vi "Import - Buffered Rx Packet.vi"(7 "Rx Packet":T2 {"targetPriority" min=-2 max=16 step=1; "targetProcessor" min=-2 max=16 step=1; "Endianness" items=["big-endian"=0, "little-endian"=2]}, 8 "error in (no error)":errorcluster, 11 "Device Item Ref in":T1 format="%.0x") -> (0 "error out":errorcluster, 3 "Device Item Ref out":T1 format="%.0x")   [LabVIEW 2019, in "UDP-Custom-Device System Explorer.lvlib"]
uses:
  UDP-Custom-Device System Explorer.lvlib
  <vilib>/NI VeriStand/Custom Device API/Custom Device Item Ref.ctl
  Types/XML - New/ImpExp - Rx Packet Data.ctl
  <vilib>/NI VeriStand/Custom Device API/Custom Device Item Info.ctl
  Shared/Types/Shared - Channel Data Type.ctl
  Shared/Types/Shared - Buffered.PacketInfo.ctl
  Shared/Types/Shared - Pointer Encoding.ctl
  Shared/Types/Shared - Receive Buffer Options.ctl
  Shared/Types/Shared - Transmit Buffer Options.ctl
  Shared/Types/Shared - New Data Options.ctl
  Shared/Types/Shared - Thread Management.ctl
  Property Accessors/Shared Packet Accessors.lvlib
  Property Accessors/Rx Packet Accessors.lvlib
  <vilib>/NI VeriStand/Custom Device API/Custom Device API.lvlib
  Property Accessors/Buffered Data Packet.lvlib
  Shared/UDP-Custom-Device Shared.lvlib
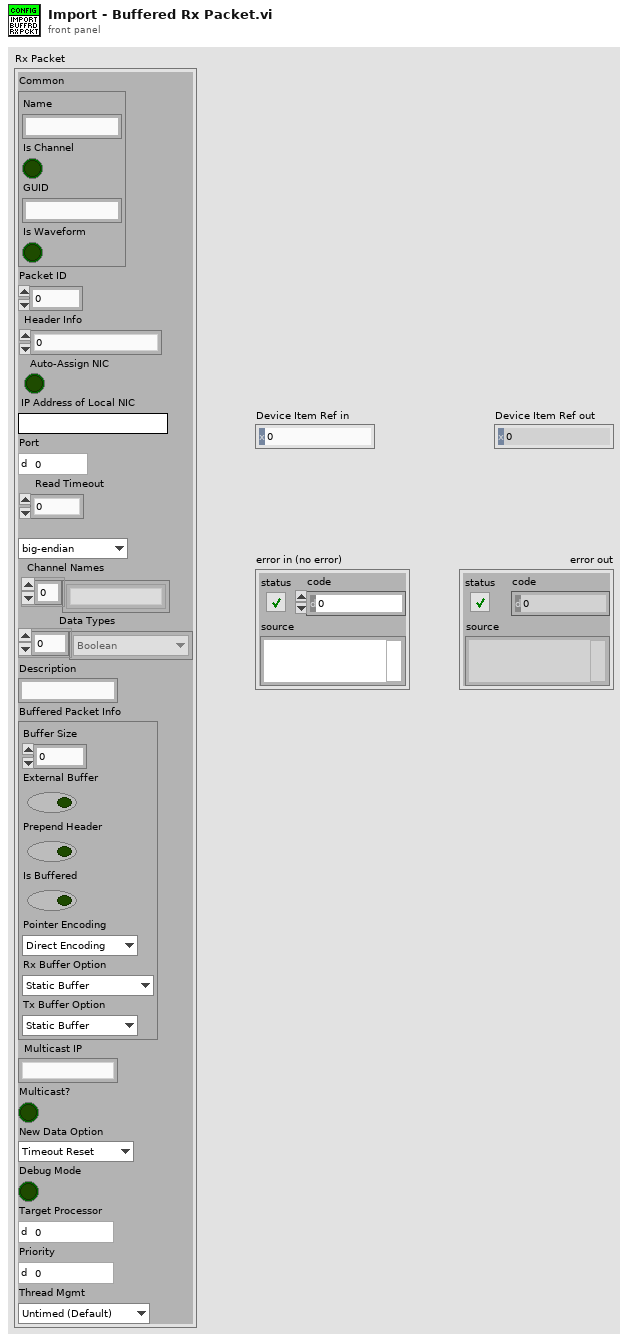
[diagram p1: front panel]
types:
  T1 = typedef "Custom Device API.lvlib/Custom Device Item Ref.ctl" = u64
  T2 = typedef "UDP-Custom-Device System Explorer.lvlib/ImpExp - Rx Packet Data.ctl" = cluster{"Common":T3, "Packet ID":i32, "Header Info":u32, "Auto-Assign NIC":bool, "IP Address of Local NIC":string, "Port":u16, "Read Timeout":i32, "Endianness":u16, "Channel Names":string[], "Data Types":T4[], "Description":string, "Buffered Packet Info":T5, "Multicast IP":string, "Multicast?":bool, "New Data Option":T9, "Debug Mode":bool, "targetProcessor":i8, "targetPriority":i16, "Thread Mgmt":T10}
  T3 = typedef "Custom Device API.lvlib/Custom Device Item Info.ctl" = cluster{"Name":string, "Is Channel":bool, "GUID":string, "Is Waveform":bool}
  T4 = typedef "UDP-Custom-Device Shared.lvlib/Shared - Channel Data Type.ctl" = enum16{"Boolean", "Single", "Double", "I8", "I16", "I32", "I64", "U8", "U16", "U32", "U64"}
  T5 = typedef "UDP-Custom-Device Shared.lvlib/Shared - Buffered.PacketInfo.ctl" = cluster{"Buffer Size":i32, "External Buffer":bool, "Prepend Header":bool, "Is Buffered":bool, "Pointer Encoding":T6, "Rx Buffer Option":T7, "Tx Buffer Option":T8}
  T6 = typedef "UDP-Custom-Device Shared.lvlib/Shared - Pointer Encoding.ctl" = enum16{"Direct Encoding", "Conversion Encoding"}
  T7 = typedef "UDP-Custom-Device Shared.lvlib/Shared - Receive Buffer Options.ctl" = enum16{"Static Buffer", "Circular Buffer", "Circular Buffer + Size", "Internal Cache", "Internal Cache + Size", "Ping Pong", "Ping Pong + Size"}
  T8 = typedef "UDP-Custom-Device Shared.lvlib/Shared - Transmit Buffer Options.ctl" = enum16{"Static Buffer", "FIFO Buffer", "FIFO Buffer + Port"}
  T9 = typedef "UDP-Custom-Device Shared.lvlib/Shared - New Data Options.ctl" = enum16{"Timeout Reset", "Counter"}
  T10 = typedef "UDP-Custom-Device Shared.lvlib/Shared - Thread Management.ctl" = enum16{"Untimed (Default)", "Timed (High Priority)"}
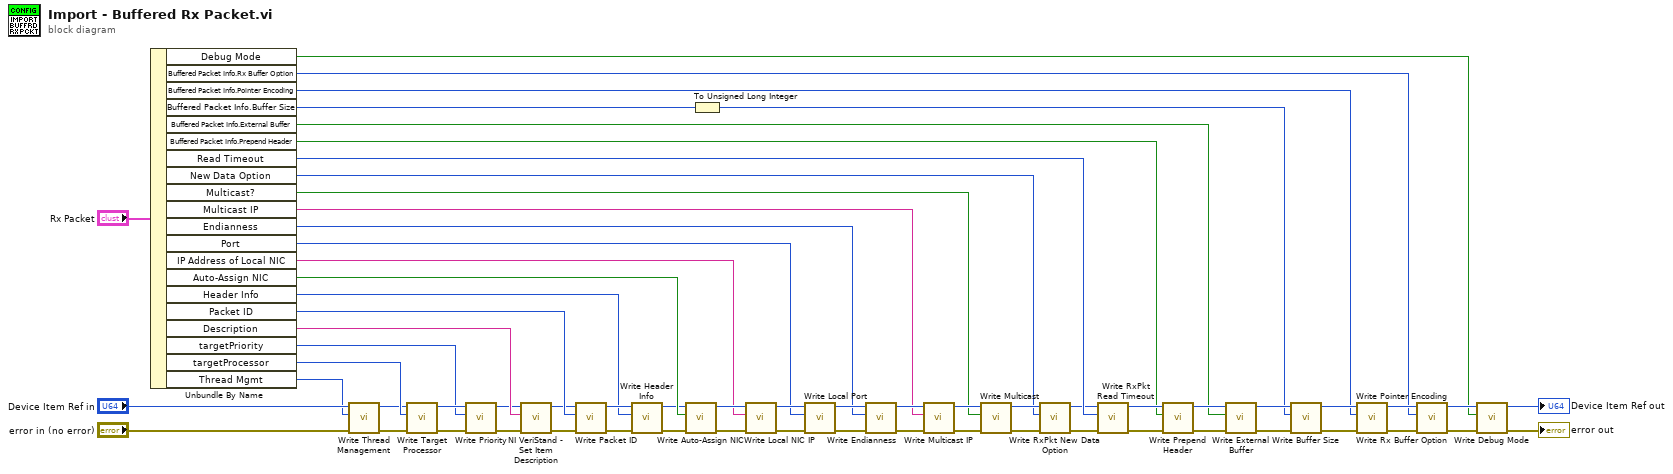
[diagram p0: block diagram]
diagram:
  n1 = Unbundle By Name("Rx Packet") -> ("Debug Mode"=w15:bool, "Buffered Packet Info.Rx Buffer Option"=w17:T7, "Buffered Packet Info.Pointer Encoding"=w25:T6, "Buffered Packet Info.Buffer Size"=w35:i32, "Buffered Packet Info.External Buffer"=w36:bool, "Buffered Packet Info.Prepend Header"=w37:bool, "Read Timeout"=w48:i32, "New Data Option"=w20:T9, "Multicast?"=w28:bool, "Multicast IP"=w29:string, "Endianness"=w49:u16, "Port"=w52:u16, "IP Address of Local NIC"=w55:string, "Auto-Assign NIC"=w59:bool, "Header Info"=w60:u32, "Packet ID"=w63:i32, "Description"=w46:string, "targetPriority"=w10:i16, "targetProcessor"=w9:i8, "Thread Mgmt"=w2:T10)
  n2 = call "Write Thread Management.vi"("error in (no error)"="error in (no error)", "Thread Management"=w2, "Node Ptr"="Device Item Ref in") -> ("error out"=w3:errorcluster, "Node Ptr out"=w5:T1)  [unwired: 7 in]
  n3 = call "Write Target Processor.vi"("error in (no error)"=w3, "targetProcessor"=w9, "Node Ptr"=w5) -> ("error out"=w11:errorcluster, "Node Ptr out"=w12:T1)  [unwired: 7 in]
  n4 = call "Write Priority.vi"("error in (no error)"=w11, "targetPriority"=w10, "Node Ptr"=w12) -> ("error out"=w8:errorcluster, "Node Ptr out"=w7:T1)  [unwired: 7 in]
  n5 = call <vilib>:"NI VeriStand - Set Item Description.vi"("error in (no error)"=w8, "Description"=w46, "Item Ref in"=w7) -> ("error out"=w44:errorcluster, "Item Ref out"=w45:T1)  [unwired: 6 in, 1 out]
  n6 = call "Write Packet ID.vi"("error in (no error)"=w44, "Packet ID"=w63, "Node Ptr"=w45) -> ("error out"=w61:errorcluster, "Node Ptr out"=w62:T1)  [unwired: 7 in]
  n7 = call "Write Header Info.vi"("error in (no error)"=w61, "Header Info"=w60, "Node Ptr"=w62) -> ("error out"=w57:errorcluster, "Node Ptr out"=w58:T1)  [unwired: 7 in]
  n8 = call "Write Auto-Assign NIC.vi"("error in (no error)"=w57, "Auto-Assign NIC"=w59, "Node Ptr"=w58) -> ("error out"=w54:errorcluster, "Node Ptr out"=w56:T1)  [unwired: 7 in]
  n9 = To Unsigned Long Integer(number=w35) -> (unsigned 32bit integer=w34:u32)
  n10 = call "Write Local NIC IP.vi"("error in (no error)"=w54, "IP Address of Local NIC"=w55, "Node Ptr"=w56) -> ("error out"=w51:errorcluster, "Node Ptr out"=w53:T1)  [unwired: 7 in]
  n11 = call "Write Local Port.vi"("error in (no error)"=w51, "Port"=w52, "Node Ptr"=w53) -> ("error out"=w47:errorcluster, "Node Ptr out"=w50:T1)  [unwired: 7 in]
  n12 = call "Write Endianness.vi"("error in (no error)"=w47, "Endianness"=w49, "Node Ptr"=w50) -> ("error out"=w30:errorcluster, "Node Ptr out"=w31:T1)  [unwired: 7 in]
  n13 = call "Write Multicast IP.vi"("error in (no error)"=w30, "Multicast IP Address"=w29, "Node Ptr"=w31) -> ("error out"=w33:errorcluster, "Node Ptr out"=w32:T1)  [unwired: 7 in]
  n14 = call "Write Multicast.vi"("error in (no error)"=w33, "Multicast"=w28, "Node Ptr"=w32) -> ("error out"=w22:errorcluster, "Node Ptr out"=w24:T1)  [unwired: 7 in]
  n15 = call "Write RxPkt New Data Option.vi"("error in (no error)"=w22, "New Data Option"=w20, "Node Ptr"=w24) -> ("error out"=w21:errorcluster, "Node Ptr out"=w23:T1)  [unwired: 7 in]
  n16 = call "Write RxPkt Read Timeout.vi"("error in (no error)"=w21, "Read Timeout"=w48, "Node Ptr"=w23) -> ("error out"=w40:errorcluster, "Node Ptr out"=w43:T1)  [unwired: 7 in]
  n17 = call "Write Prepend Header.vi"("error in (no error)"=w40, "Prepend Header"=w37, "Node Ptr"=w43) -> ("error out"=w39:errorcluster, "Node Ptr out"=w42:T1)  [unwired: 7 in]
  n18 = call "Write External Buffer.vi"("error in (no error)"=w39, "External Buffer"=w36, "Node Ptr"=w42) -> ("error out"=w38:errorcluster, "Node Ptr out"=w41:T1)  [unwired: 7 in]
  n19 = call "Write Buffer Size.vi"("error in (no error)"=w38, "Buffer Size"=w34, "Node Ptr"=w41) -> ("error out"=w27:errorcluster, "Node Ptr out"=w26:T1)  [unwired: 7 in]
  n20 = call "Write Pointer Encoding.vi"("error in (no error)"=w27, "Pointer Encoding"=w25, "Node Ptr"=w26) -> ("error out"=w19:errorcluster, "Node Ptr out"=w18:T1)  [unwired: 7 in]
  n21 = call "Write Rx Buffer Option.vi"("error in (no error)"=w19, "Buffer Option"=w17, "Node Ptr"=w18) -> ("error out"=w14:errorcluster, "Node Ptr out"=w16:T1)  [unwired: 7 in]
  n22 = call "Write Debug Mode.vi"("error in (no error)"=w14, "Debug Mode"=w15, "Node Ptr"=w16) -> ("error out"=→"error out":errorcluster, "Node Ptr out"=→"Device Item Ref out":T1)  [unwired: 7 in]
